vi "Create Laplacian 32f.vi"(8 "Error In":errorcluster, 9 "Dimension":T1={"Depth"=1, "Height"=1, "Width"=1} {"Width" min=1; "Height" min=1; "Depth" min=1}, 10 "Memory Object":T2 {"Dimension"."Width" min=1; "Dimension"."Height" min=1; "Dimension"."Depth" min=1}, 11 "Device In":T3) -> (0 "Error Out":errorcluster, 1 "Dimension Out":T1={"Depth"=1, "Height"=1, "Width"=1} {"Width" min=1; "Height" min=1; "Depth" min=1}, 3 "Laplacian Out":T6 {"Laplacian Out"."Dimension"."Width" min=1; "Laplacian Out"."Dimension"."Height" min=1; "Laplacian Out"."Dimension"."Depth" min=1})   [LabVIEW 2012, in "OpenCLV x64.lvlib"]
doc: "Creates a Laplacian Object and allocates space for the destination memory object. Either the dimension or a prior memory object must be provided."
uses:
  OpenCLV x64.lvlib
  Controls/Device ID.ctl
  User Controls/Array Dimensions.ctl
  Controls/Laplacian Object.ctl
  Controls/Program Handle.ctl
  Controls/Memory Object.ctl
  Controls/Memory ID.ctl
  Controls/Memory Type.ctl
  Allocate Memory/AllocateMemory_32f.vi
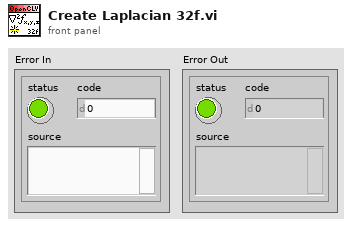
[diagram p1: front panel]
types:
  T1 = typedef "Array Dimensions.ctl" = cluster{"Depth":u64, "Height":u64, "Width":u64}
  T2 = typedef "OpenCLV x64.lvlib/Memory Object.ctl" = cluster{"Device ID":T3, "Memeroy ID":T4, "Dimension":T1, "Memory Type":T5}
  T3 = typedef "OpenCLV x64.lvlib/Device ID.ctl" = u64
  T4 = typedef "OpenCLV x64.lvlib/Memory ID.ctl" = u64
  T5 = typedef "OpenCLV x64.lvlib/Memory Type.ctl" = enum16{"32f", "u8", "i8", "u16", "i16", "u32", "i32", "64f"}
  T6 = typedef "OpenCLV x64.lvlib/Laplacian Object.ctl" = cluster{"Device Out":T3, "Program Handle":T7, "Laplacian Out":T2}
  T7 = typedef "OpenCLV x64.lvlib/Program Handle.ctl" = u64
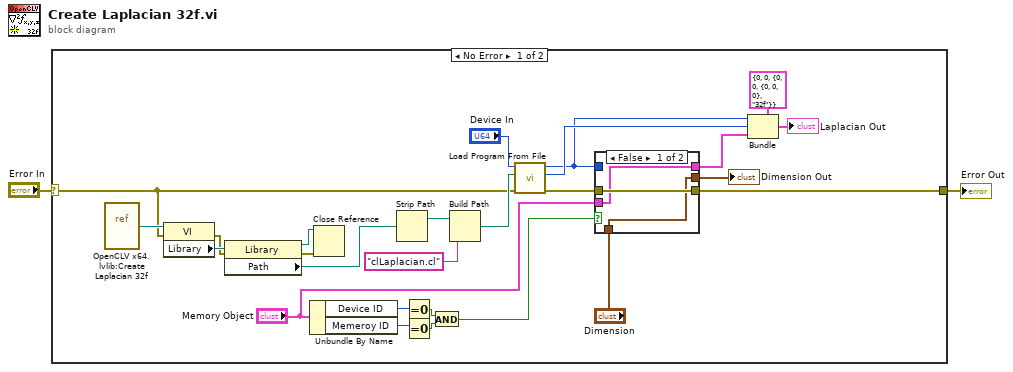
[diagram p0: block diagram]
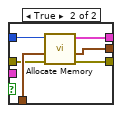
[diagram p2: hidden frame]
diagram:
  n1 = case shown="No Error" "Error In" {
    selector: "Error In" -> [w3 w38]
    tunnel: [w6 w38] -> w1
    frame No Error {
      n2 = vi-ref "OpenCLV x64.lvlib:Create Laplacian 32f.vi"() -> (w22:refnum<vi>)
      n3 = property class="VI"(reference=w22, error in=w3) -> (error out=w4:errorcluster, "Library"=w21:refnum<vi>)  [unwired: 1 out]
      n4 = property class="Library"(reference=w21, error in=w4) -> (reference out=w7:refnum<vi>, error out=w8:errorcluster, "Path"=w20:path)
      n5 = Unbundle By Name("Memory Object") -> ("Device ID"=w13:T3, "Memeroy ID"=w14:T4)
      n6 = Close Reference(reference=w7, error in (no error)=w8) -> ()  [unwired: 1 out]
      n7 = Strip Path(path=w20) -> (stripped path=w28:path)  [unwired: 1 out]
      n8 = Equal To 0?(x=w13) -> (x = 0?=w11:bool)
      n9 = Equal To 0?(x=w14) -> (x = 0?=w12:bool)
      n10 = And(x=w11, y=w12) -> (x .and. y?=w10:bool)
      n11 = Build Path(base path=w28, name or relative path="clLaplacian.cl") -> (appended path=w26:path)
      n12 = call "Load Program From File.vi"("Error In"=w3, "Program Path"=w26, "Device In"="Device In") -> ("Error Out"=w23:errorcluster, "Program Handle"=w16:T7, "Device Out"=w15:T3)  [unwired: 6 in]
      n13 = case shown="False" w10 {
        tunnel: "Dimension" -> [w29 w37]
        tunnel: w23 -> [w31 w36]
        tunnel: [w30 w35] -> w19
        tunnel: [w31 w34] -> w6
        tunnel: w15 -> [_ w33]
        tunnel: "Memory Object" -> [w30 _]
        tunnel: [w29 w32] -> w5
        frame False {
        }
        frame True {
          n14 = call-poly "Allocate Memory.vi"("Error In"=w36, "Dimension"=w37, "Device In"=w33) -> ("Error Out"=w34:errorcluster, "Dimension Out"=w32:T1, "Memory Object"=w35:T2)  [unwired: 6 in]
        }
      }
      "Dimension Out" <- w5
      n15 = Bundle(cluster=T6 {"Device Out"=0, "Program Handle"=0, "Laplacian Out"={"Device ID"=0, "Memeroy ID"=0, "Dimension"={"Depth"=0, "Height"=0, "Width"=0}, "Memory Type"=enum."32f"}} ("Laplacian Object"), "Device Out"=w15, "Program Handle"=w16, "Laplacian Out"=w19) -> (→"Laplacian Out":T6)
    }
    frame Error {
    }
  }
  "Error Out" <- w1
